vi "RSZVB Set PI Controller Gain.vi"(7 "Gain (0.4)":dbl=0.4 format="%^.3e", 8 "error in (no error)":errorcluster {"code" format="%.0x"}, 9 "Port (1)":i32=1, 10 "Channel (1)":i32=1, 11 "VISA session":refnum<visa-resource-name>) -> (0 "error out":errorcluster {"code" format="%.0x"}, 3 "dup VISA session":refnum<visa-resource-name>)   [LabVIEW 2011]
doc: "Defines the proportional gain of the PI controller at source port <Pt>. This setting takes effect when manual setting of the controller parameters is enabled. \n\nRemote-control command(s):\nSOURce<Ch>:POWer<Pt>:ALC:PIParameter:GAIN"
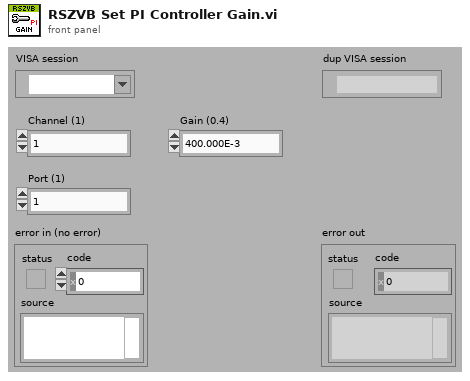
[diagram p1: front panel]
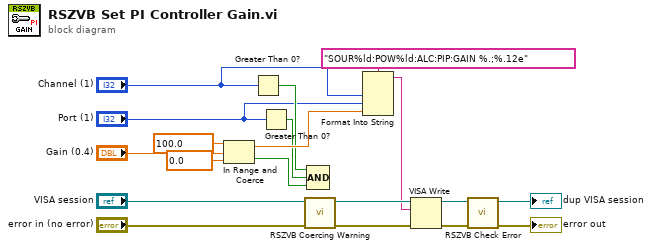
[diagram p0: block diagram]
diagram:
  n1 = In Range and Coerce(upper limit=100.0, x="Gain (0.4)", lower limit=0.0) -> (coerced(x)=w11:dbl, In Range?=w10:bool)
  n2 = Greater Than 0?(x="Channel (1)") -> (x > 0?=w8:bool)
  n3 = Greater Than 0?(x="Port (1)") -> (x > 0?=w9:bool)
  n4 = call "RSZVB Coercing Warning.vi"("error in (no error)"="error in (no error)", "VISA session"="VISA session") -> ("error out"=w17:errorcluster, "dup VISA session"=w18:refnum<visa-resource-name>)  [unwired: 8 in]
  n5 = Compound Arithmetic op=AND(w8, w9, w10) -> ()  [unwired: 1 out]
  n6 = Format Into String(format string="SOUR%ld:POW%ld:ALC:PIP:GAIN %.;%.12e", "Channel (1)", "Port (1)", w11) -> (resulting string=w14:string)  [unwired: 2 in, 1 out]
  n7 = VISA Write(VISA resource name=w18, write buffer=w14, error in (no error)=w17) -> (VISA resource name out=w15:refnum<visa-resource-name>, error out=w16:errorcluster)  [unwired: 1 out]
  n8 = call "RSZVB Check Error.vi"("error in (no error)"=w16, "VISA session"=w15) -> ("error out"=→"error out":errorcluster, "dup VISA session"=→"dup VISA session":refnum<visa-resource-name>)  [unwired: 8 in]
